vi "Get Minimal Maximal Size.vi"(7 "Vertical? [F, hor.]":bool, 8 "error in (no error)":errorcluster, 11 "IObject in":refnum<class "IObject.lvclass">) -> (0 "error out":errorcluster, 1 "Minimal size":i16, 2 "Maximal size":i16, 3 "IObject out":refnum<class "IObject.lvclass">)   [LabVIEW 2013, in "IObject.lvclass"]
uses:
  IObject.lvclass
  IObject.lvclass/IObject.ctl
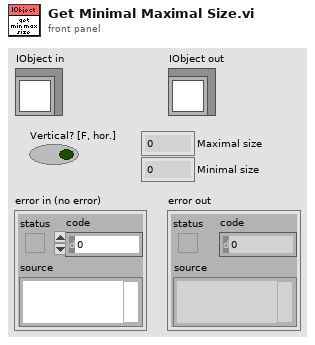
[diagram p1: front panel]
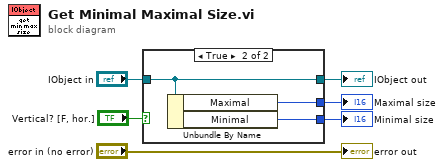
[diagram p0: block diagram]
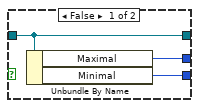
[diagram p2: hidden frame]
diagram:
  n1 = case shown="True" "Vertical? [F, hor.]" {
    tunnel: "IObject in" -> [w7 w10]
    tunnel: [w9 w12] -> w4
    tunnel: [w8 w11] -> w3
    tunnel: [w7 w10] -> w2
    frame False {
      n2 = Unbundle By Name(w7) -> ("Maximal"=w9:i16, "Minimal"=w8:i16)
    }
    frame True {
      n3 = Unbundle By Name(w10) -> ("Maximal"=w12:i16, "Minimal"=w11:i16)
    }
  }
  "IObject out" <- w2
  "Maximal size" <- w4
  "Minimal size" <- w3
  "error out" <- "error in (no error)"
